vi "niFPGA Discrete Delay.vi"(0 "initial condition":i32, 2 "input":i32, 5 "initialize":bool) -> (7 "output":i32)   [LabVIEW 2020]
doc: "Delays the input value for the number of loop iterations you specify in the <B>Configure Basic Discrete Delay</B> dialog box."
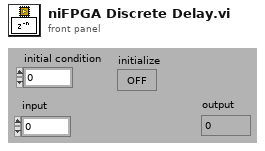
[diagram p1: front panel]
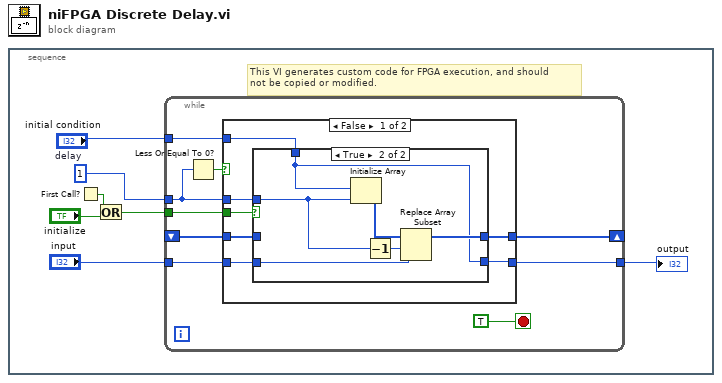
[diagram p0: block diagram]
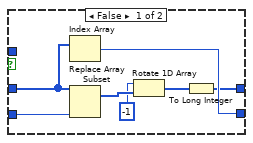
[diagram p2: hidden frame]
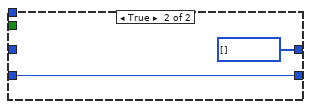
[diagram p3: hidden frame]
diagram:
  n1 = stacked-sequence {
    frame #0 {
      w6 = u8 1  # delay
      # "This VI generates custom code for FPGA execution, and should\nnot be copied or modified."
      n2 = First Call?() -> (First Call?: T/F=w2:bool)
      n3 = Or(x=w2, y="initialize") -> (x .or. y?=w1:bool)
      n4 = while {
        tunnel: "input" -> [w14]
        shift-left: _ -> [w10]
        shift-right: [w15] -> _
        tunnel: w6 -> [w12]
        tunnel: w1 -> [w16]
        tunnel: "initial condition" -> [w9]
        tunnel: [w8] -> w3
        stop <- TRUE stop-if-true
        n5 = Less Or Equal To 0?(x=w12) -> (x <= 0?=w11:bool)
        n6 = case shown="False" w11 {
          tunnel: w16 -> [w23 _]
          tunnel: w12 -> [w22 _]
          tunnel: [w21 i32[] []] -> w15
          tunnel: w10 -> [w20 _]
          tunnel: w14 -> [w19 w38]
          tunnel: [w18 w38] -> w8
          tunnel: w9 -> [w17 _]
          frame False {
            n7 = case shown="True" w23 {
              tunnel: w22 -> [_ w33]
              tunnel: [w27 w35] -> w21
              tunnel: w20 -> [w29 _]
              tunnel: w19 -> [w30 w34]
              tunnel: [w28 w31] -> w18
              tunnel: w17 -> [_ w31]
              frame False {
                n8 = Index Array(array=w29) -> (element=w28:i32)  [unwired: 1 in]
                n9 = Replace Array Subset(array=w29, new element=w30) -> (w26:i32[])  [unwired: 1 in]
                n10 = Rotate 1D Array(1:w26, 2:-1 ("n")) -> (0:w25:i32[])
                n11 = To Long Integer(number=w25) -> (32bit integer=w27:i32[])
              }
              frame True {
                n12 = Initialize Array(w31, w33) -> (w36:i32[])
                n13 = Decrement(x=w33) -> (x-1=w32:u8)
                n14 = Replace Array Subset(array=w36, new element=w34, index=w32) -> (w35:i32[])
              }
            }
          }
          frame True {
          }
        }
      }
      "output" <- w3
    }
  }
